vi "Up_Overlay Pattern Matching.vi"(6 "Color":u32(colorbox)=16711680, 7 "Group":string, 8 "error in":errorcluster, 10 "Matches":T2(array[cluster]), 11 "Image":T1) -> (0 "error out":errorcluster, 3 "Image Out":T1)   [LabVIEW 2019]
uses:
  <vilib>/vision/Image Controls.llb/IMAQ Image.ctl
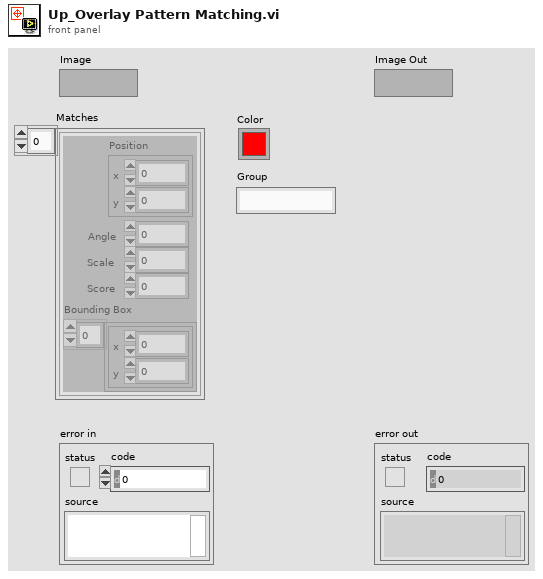
[diagram p1: front panel]
types:
  T1 = typedef "IMAQ Image.ctl" = refnum<image>
  T2 = cluster{"Position":cluster{"x":sgl, "y":sgl}, "Angle":sgl, "Scale":sgl, "Score":sgl, "Bounding Box":cluster{"x":sgl, "y":sgl}[]}[]
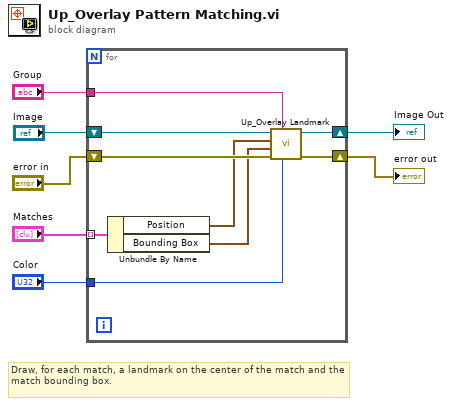
[diagram p0: block diagram]
diagram:
  # "Draw, for each match, a landmark on the center of the match and the match bounding box."
  n1 = for {
    shift-right: [w13] -> w6
    shift-left: "Image" -> [w15]
    tunnel: "Matches" -> [w16] mode=indexing
    tunnel: "Color" -> [w8]
    shift-right: [w11] -> w2
    shift-left: "error in" -> [w12]
    tunnel: "Group" -> [w14]
    n2 = Unbundle By Name(w16) -> ("Position"=w10:cluster{"x":sgl, "y":sgl}, "Bounding Box"=w9:cluster{"x":sgl, "y":sgl}[])
    n3 = call "Up_Overlay Landmark.vi"("Color"=w8, "Group"=w14, "error in"=w12, "Bounding Box"=w9, "Position"=w10, "Image"=w15) -> ("error out"=w11:errorcluster, "Image Out"=w13:T1)  [unwired: 4 in]
  }
  "Image Out" <- w6
  "error out" <- w2
